vi "Load Store Sweep List.vi"(7 "Operation Type (0: Load)":i32(ring) items=["Load", "Store"], 8 "error in (no error)":errorcluster, 9 "File Name":string, 10 "Channel (1: Channel 1)":i32(ring)=1 items=["Channel 1"=1], 11 "VISA resource name":refnum<visa-resource-name>) -> (0 "error out":errorcluster, 3 "VISA resource name out":refnum<visa-resource-name>)   [LabVIEW 2012, in "Keysight B2980 Series.lvlib"]
doc: "Loads or stores a list sweep data from or to the specified file in the current directory."
uses:
  Keysight B2980 Series.lvlib
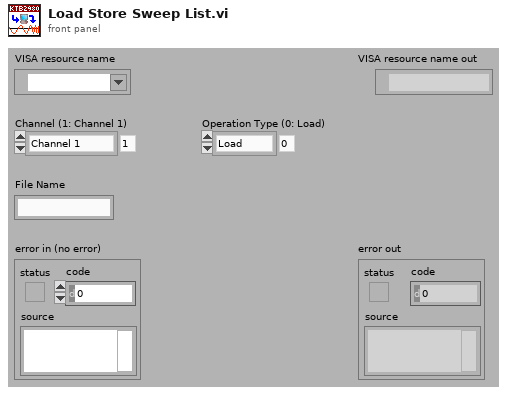
[diagram p1: front panel]
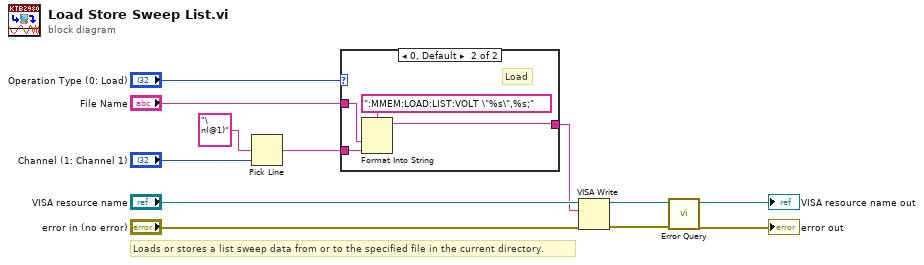
[diagram p0: block diagram]
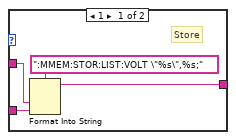
[diagram p2: hidden frame]
diagram:
  # "Loads or stores a list sweep data from or to the specified file in the current directory."
  n1 = Pick Line(multi-line string="\n(@1)", line index="Channel (1: Channel 1)") -> (output string=w6:string)  [unwired: 1 out]
  n2 = case shown="0, Default" "Operation Type (0: Load)" {
    tunnel: "File Name" -> [w15 w19]
    tunnel: [w14 w18] -> w1
    tunnel: w6 -> [w13 w17]
    frame 1 {
      # "Store"
      n3 = Format Into String(format string=":MMEM:STOR:LIST:VOLT \"%s\",%s;", w15, w13) -> (resulting string=w14:string)  [unwired: 2 in, 1 out]
    }
    frame 0, Default {
      # "Load"
      n4 = Format Into String(format string=":MMEM:LOAD:LIST:VOLT \"%s\",%s;", w19, w17) -> (resulting string=w18:string)  [unwired: 2 in, 1 out]
    }
  }
  n5 = VISA Write(VISA resource name="VISA resource name", write buffer=w1, error in (no error)="error in (no error)") -> (VISA resource name out=w5:refnum<visa-resource-name>, error out=w4:errorcluster)  [unwired: 1 out]
  n6 = call "Error Query.vi"("error in (no error)"=w4, "VISA resource name"=w5) -> ("error out"=→"error out":errorcluster, "VISA resource name out"=→"VISA resource name out":refnum<visa-resource-name>)  [unwired: 8 out]
